vi "Cache-Broadcast Registry Search Result.vi"(8 "error in (no error)":errorcluster, 10 "CSM Name":string, 11 "Broadcast State":string) -> (0 "error out":errorcluster, 3 "Array":T2(array[cluster]))   [LabVIEW 2017, in "Communicable State Machine.lvlib"]
doc: "### Cache-Broadcast Registry Search Result.vi\n\n-- <b>Controls</b> --\n- <b>CSM Name</b>:\n- <b>Broadcast state</b>:\n\n-- <b>Indicators</b> --\n- <b>Array</b>:"
uses:
  AdvanceAPI/CSM - Broadcast Message Type.ctl
  Typedef/_CSM_List Module Scope.ctl
  Operation-BroadcastRegistry.ctl
  ChangeFlag/ChangeFlag-Read.vi
  ChangeFlag/ChangeFlagDB.vi
  Communicable State Machine.lvlib
  _Shared/CSM Shared.lvlib
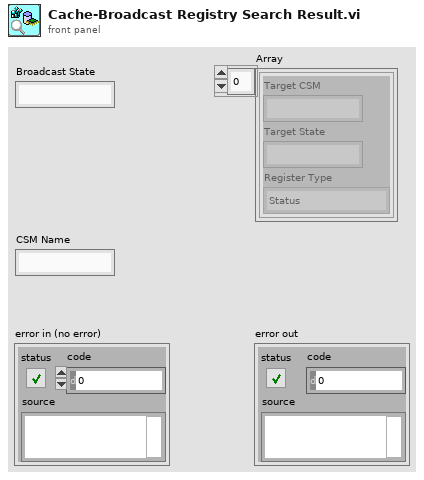
[diagram p1: front panel]
types:
  T1 = typedef "Communicable State Machine.lvlib/CSM - Broadcast Message Type.ctl" = enum16{"<Null>", "Status", "Interrupt"}
  T2 = cluster{"Target CSM":string, "Target State":string, "Register Type":T1}[]
  T3 = cluster{"Target CSM":string, "Target State":string, "Register Type":T1}
  T4 = typedef "Communicable State Machine.lvlib/_CSM_List Module Scope.ctl" = enum16{"Normal", "System Only", "All"}
  T5 = typedef "Communicable State Machine.lvlib/Operation-BroadcastRegistry.ctl" = enum16{"Delete Source Module", "Delete Target Module", "Remove Module", "Register", "Unregister", "Check", "List Status", "List Entries", "List Status Of Source", "Drop", "Register As Status", "Register As Interrupt"}
  T6 = typedef "Communicable State Machine.lvlib/BroadcastRegistry-Value.ctl" = cluster{"Name":string, "Register Type":T1}
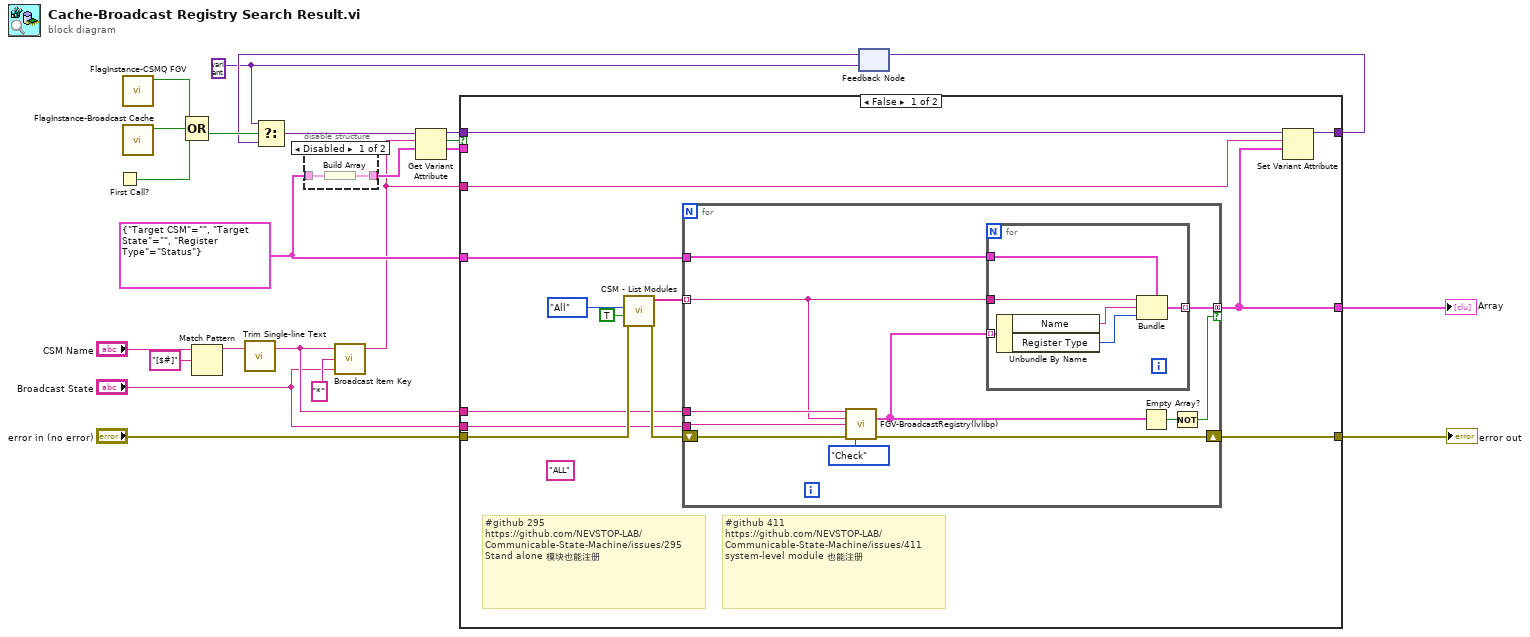
[diagram p0: block diagram]
diagram:
  w15 = T3 {"Target CSM"="", "Target State"="", "Register Type"=enum."Status"} ("cluster")
  w17 = variant
  n1 = First Call?() -> (First Call?: T/F=w20:bool)
  n2 = call "FlagInstance-CSMQ FGV.vi"() -> ("Changed"=w2:bool)  [unwired: 10 in, 1 out]
  n3 = call "FlagInstance-Broadcast Cache.vi"() -> ("Changed"=w1:bool)  [unwired: 10 in, 1 out]
  n4 = Compound Arithmetic op=OR(w2, w1, w20) -> (w19:bool)
  n5 = Match Pattern(string="CSM Name", regular expression="[$#]") -> (before substring=w8:string)  [unwired: 1 in, 3 out]
  n6 = call "Trim Single-line Text.vi"("single-line text"=w8) -> ("trimed text"=w6:string)  [unwired: 2 in]
  n7 = disable-structure shown="Disabled" {
    disable-tunnel: w15 -> [w25 _]
    disable-tunnel: [w24 _] -> w14
    frame Disabled {
      n8 = Build Array(w25) -> (w24:T2)
    }
    frame Enabled {
    }
  }
  n9 = call "Broadcast Item Key.vi"("Status"="Broadcast State", "Target"="*" ("target"), "Source"=w6) -> ("Key"=w3:string)  [unwired: 2 in]
  n10 = feedback #1(w17) -> (w18:variant)
  n11 = Select(t=w17, s=w19, f=w18) -> (s? t:f=w16:variant)
  n12 = Get Variant Attribute(Variant=w16, name=w3, default value (empty Variant)=w14) -> (duplicate Variant=w12:variant, found=w13:bool, value=w11:T2)  [unwired: 1 in, 1 out]
  n13 = case shown="False" w13 {
    tunnel: [w38 w57] -> w23
    tunnel: "error in (no error)" -> [w36 w57]
    tunnel: [w30 w58] -> w21
    tunnel: "Broadcast State" -> [w35 _]
    tunnel: w6 -> [w34 _]
    tunnel: w15 -> [w33 _]
    tunnel: w12 -> [w32 w56]
    tunnel: w11 -> [_ w58]
    tunnel: w3 -> [w31 _]
    tunnel: [w29 w56] -> w10
    frame False {
      (unwired) "ALL" ("Name (\"\" to Use UUID) in")
      # "#github 411\nhttps://github.com/NEVSTOP-LAB/Communicable-State-Machine/issues/411\nsystem-level module 也能注册"
      # "#github 295\nhttps://github.com/NEVSTOP-LAB/Communicable-State-Machine/issues/295\nStand alone 模块也能注册"
      n14 = call "CSM - List Modules.vi"("Error In"=w36, "With Nodes? (F)"=TRUE ("With Instance(F)"), "Scope (Normal)"=_CSM_List_Module_Scope."All" ("Scope(Normal)")) -> ("error out"=w37:errorcluster, "Module Names"=w28:string[])  [unwired: 7 in]
      n15 = for {
        tunnel: w34 -> [w47]
        tunnel: w35 -> [w44]
        shift-right: [w46] -> w38
        shift-left: w37 -> [w48]
        tunnel: [w43] -> w30 mode=concatenating if=w45
        tunnel: w33 -> [w42]
        tunnel: w28 -> [w40] mode=indexing
        n16 = call "FGV-BroadcastRegistry(lvlibp).vi"("Source"=w47, "Target"=w40, "Status"=w44, "Error In"=w48, "Operation"=Operation-BroadcastRegistry."Check") -> ("Values"=w39:T6[], "error out"=w46:errorcluster)  [unwired: 8 in, 1 out]
        n17 = for {
          tunnel: w40 -> [w53]
          tunnel: w42 -> [w54]
          tunnel: [w55] -> w43 mode=indexing
          tunnel: w39 -> [w52] mode=indexing
          n18 = Unbundle By Name(w52) -> ("Name"=w51:string, "Register Type"=w50:T1)
          n19 = Bundle(cluster=w54, "Target CSM"=w53, "Target State"=w51, "Register Type"=w50) -> (w55:T3)
        }
        n20 = Empty Array?(array=w39) -> (empty?=w41:bool)
        n21 = Not(x=w41) -> (.not. x?=w45:bool)
      }
      n22 = Set Variant Attribute(Variant=w32, name=w31, value=w30) -> (Variant out=w29:variant)  [unwired: 1 in, 2 out]
    }
    frame True {
    }
  }
  "error out" <- w23
  "Array" <- w21
  n23 = feedback-in #1(w10) -> ()
